vi "example_3_5_c.vi"() -> ()   [LabVIEW 2018]
panel:
  in  "stop":bool
  out "Boolean":bool
  in  "BLUE":u32
  in  "GREEN":u32
  in  "RED":u32
  # "NOTE: remember plug the Led Analyser\nbefore run LabVIEW and to change the\nVISA resource name in the schematic,\notherwise the application will not work."
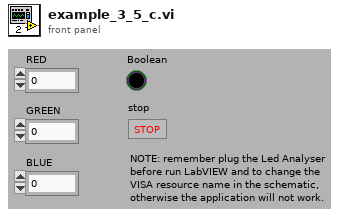
[diagram p1: front panel]
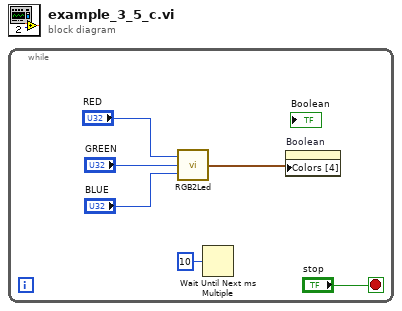
[diagram p0: block diagram]
diagram:
  n1 = while {
    stop <- "stop" stop-if-true
    n2 = call "RGB2Led.vi"("B"="BLUE", "G"="GREEN", "R"="RED") -> ("Colors [4]"=w2:cluster{u32, u32}[])
    n3 = Wait Until Next ms Multiple(millisecond multiple=u32 10) -> ()  [unwired: 1 out]
    n4 = property on="Boolean" class="Bool (strict)"("Colors [4]"=w2) -> ()  [unwired: 2 in, 2 out]
  }
